vi "UHR-Fleezers Control (host) -TL FB Corrected Ronen semipassive - stepping.vi"(0 "Tab Control":T5(tab)=enum."Trap Control (RF)") -> ()   [LabVIEW 2013] (continued)
        n480 = xnode "Read/Write Control"("FPGA VI Reference In"=w830, "error in"=w829, "Phase count adjustment"=w826) -> ("FPGA VI Reference Out"=w825:T20, "error out"=w824:errorcluster)
        n481 = Or(x="- phase (AI1)", y="+ phase (AI1)") -> (x .or. y?=w821:bool)
        n482 = xnode "Read/Write Control"("FPGA VI Reference In"=w825, "error in"=w824, "+ phase"=w821) -> ("error out"=w820:errorcluster)  [unwired: 1 out]
      }
      event "Signals to Plot": Double Click {
        w833 = u32 9868950 ("Color Box")
        n483 = event-data() -> ("Row"=w835:i32)  [unwired: 9 out]
        n484 = property on="All Signals" class="WFChart (strict)"("Active Plot"=w835) -> (error out=w846:errorcluster)  [unwired: 2 in, 1 out]
        n485 = property on="All Signals" class="WFChart (strict)" props=["Plot", "Visible?", "Plot", "Plot Color"](error in=w846) -> (error out=w845:errorcluster, "Plot.Visible?"=w844:bool)  [unwired: 1 in, 2 out]
        n486 = Select(t=FALSE ("Plot.Visible"), s=w844, f=TRUE ("Plot.Visible")) -> (s? t:f=w839:bool)
        n487 = property on="All Signals" class="WFChart (strict)"(error in=w845, "Plot.Visible?"=w839) -> (error out=w841:errorcluster)  [unwired: 1 in, 1 out]
        n488 = property on="All Signals" class="WFChart (strict)"(error in=w841) -> (error out=w836:errorcluster, "Plot.Plot Color"=w840:u32)  [unwired: 1 in, 1 out]
        n489 = property on="Signals to Plot" class="LstBox (strict)"(error in=w836, "Active Row"=w835) -> (error out=w834:errorcluster)  [unwired: 1 in, 1 out]
        n490 = Select(t=w840, s=w839, f=u32 0) -> (s? t:f=w837:u32)
        n491 = property on="Signals to Plot" class="LstBox (strict)"(error in=w834, "CellFontColor"=w837, "SelColor"=w833, "CellBG"=w833, "CellFontSize"=u32 20 ("Active Row:Cell Font:Size"), "CellFontBold"=TRUE ("Active Row:Cell Font:Bold")) -> ()  [unwired: 1 in, 2 out]
      }
      event "Dynamic Force FB": Value Change {
        n492 = event-data() -> ()  [unwired: 7 out]
        n493 = xnode "Read/Write Control"("FPGA VI Reference In"=w848, "Dynamic Force FB (Ronen)"="Dynamic Force FB") -> ()  [unwired: 1 in, 2 out]
      }
      event "BD 1 Frequency 1 (MHz)", "BD 1 Frequency 2 (MHz)", "BD 1 Frequency 3 (MHz)", "BD 2 Frequency 1 (MHz)", "BD 2 Frequency 2 (MHz)", "BD 2 Frequency 3 (MHz)", "Trap Delta (MHz)": Value Change {
        # "anytime one of the frequencies is changed, write it to the RF board UNLESS Set 2 is being oscillated. The oscillation\nscript writes the frequencies to the RF board."
        n494 = event-data() -> ("CtlRef"=w851:refnum<vi>)  [unwired: 6 out]
        n495 = control-ref of="Trap Delta (MHz)"() -> (w850:refnum<vi>)
        n496 = Equal?(x=w850, y=w851) -> (x = y?=w849:bool)
        n497 = case shown="False" "Oscillate Set 2" {
          tunnel: w854 -> [w875 _]
          tunnel: [w874 w887] -> w853
          tunnel: w852 -> [w873 w887]
          tunnel: w849 -> [w860 _]
          frame False {
            n498 = case shown="False" "Symmetric manual \ntrap motion" {
              tunnel: [w880 w886] -> w861
              tunnel: "Trap Delta (MHz)" -> [w879 w885]
              tunnel: [w878 w882] -> w857
              frame False {
                w880 = 90.0
                n499 = Subtract(x=w880, y=w879) -> (x-y=w878:dbl)
              }
              frame True {
                w881 = 80
                n500 = Divide(x=w885, y=2) -> (x/y=w883:dbl)
                n501 = Subtract(x=w881, y=w883) -> (x-y=w882:dbl)
                n502 = Add(x=w881, y=w883) -> (x+y=w886:dbl)
              }
            }
            n503 = local read "BD 1 Frequency 2 (MHz)"() -> (w862:dbl)
            n504 = local write "BD 1 Frequency 1 (MHz)"(w857) -> ()
            n505 = Select(t=w861, s=w860, f=w862) -> (s? t:f=w859:dbl)
            n506 = local read "Y RF Frequency Limits (MHz)"() -> (w863:T17)
            n507 = local read "X RF Frequency Limits (MHz)"() -> (w864:T17)
            n508 = local read "BD 1 Frequency 3 (MHz)"() -> (w876:dbl)
            n509 = local write "BD 1 Frequency 2 (MHz)"(w859) -> ()
            n510 = local read "BD 2 Frequency 1 (MHz)"() -> (w867:dbl)
            n511 = local read "BD 2 Frequency 2 (MHz)"() -> (w866:dbl)
            n512 = local read "BD 2 Frequency 3 (MHz)"() -> (w877:dbl)
            n513 = call "set RF board frequency - interlace.vi"("Board 2 Frequency Limits"=w863, "Board 1 Frequency Limits"=w864, "error in"=w873, "FPGA VI Reference In"=w875, "Board 2 Frequency 3 (MHz)"=w877, "Board 1 Frequency 3 (MHz)"=w876, "Board 2 Frequency 2 (MHz)"=w866, "Board 2 Frequency 1 (MHz)"=w867, "Board 1 Frequency 2 (MHz)"=w859, "Board 1 Frequency 1  (MHz)"=w857) -> ("error out"=w874:errorcluster)  [unwired: 1 out]
            n514 = Subtract(x=w867, y=w866) -> (x-y=w871:dbl)
            n515 = Subtract(x=w859, y=w857) -> (x-y=w872:dbl)
            n516 = Square(x=w871) -> (x^2=w869:dbl)
            n517 = Square(x=w872) -> (x^2=w870:dbl)
            n518 = Add(x=w870, y=w869) -> (x+y=w868:dbl)
            n519 = Square Root(x=w868) -> (sqrt(x)=w865:dbl)
            n520 = local write "Trap Delta (MHz)"(w865) -> ()
            n521 = property on="Initial delta (MHz)" class="DigNum (strict)"("Val(Sgnl)"=w865) -> ()  [unwired: 2 in, 2 out]
          }
          frame True {
          }
        }
      }
      event "Round T1 X": Value Change {
        n522 = event-data() -> ()  [unwired: 7 out]
        n523 = local read "BD 1 Frequency 1 (MHz)"() -> (w890:dbl)
        n524 = Round To Nearest(number=w890) -> (nearest integer value=w889:dbl)
        n525 = property on="BD 1 Frequency 1 (MHz)" class="DigNum (strict)"("Val(Sgnl)"=w889) -> ()  [unwired: 2 in, 2 out]
      }
      event "Restart RF": Value Change {
        n526 = event-data() -> ()  [unwired: 7 out]
        n527 = xnode "Read/Write Control"("FPGA VI Reference In"=w928, "error in"=w923, "FPGA Controls  RF Box"=FALSE) -> ("FPGA VI Reference Out"=w927:T20, "error out"=w922:errorcluster)
        n528 = local read "Y RF Amplitude Limits (%)"() -> (w903:T17)
        n529 = local read "X RF Amplitude Limits (%)"() -> (w904:T17)
        n530 = local read "X RF Frequency Limits (MHz)"() -> (w906:T17)
        n531 = local read "Y RF Frequency Limits (MHz)"() -> (w905:T17)
        n532 = xnode "Read/Write Control"("FPGA VI Reference In"=w927, "error in"=w922, "Direct RF Box  Communication"=TRUE) -> ("FPGA VI Reference Out"=w926:T20, "error out"=w921:errorcluster)
        n533 = local read "BD 2 Frequency 3 (MHz)"() -> (w913:dbl)
        n534 = local read "BD 2 Frequency 2 (MHz)"() -> (w914:dbl)
        n535 = local read "BD 1 Frequency 3 (MHz)"() -> (w917:dbl)
        n536 = local read "BD 1 Frequency 1 (MHz)"() -> (w918:dbl)
        n537 = local read "BD 2 Frequency 1 (MHz)"() -> (w915:dbl)
        n538 = local read "BD 1 Frequency 2 (MHz)"() -> (w916:dbl)
        n539 = call "Initialize RF boards - interlace 3.vi"("error in"=w921, "FPGA VI Reference In"=w926) -> ("error out"=w920:errorcluster, "FPGA VI Reference Out"=w925:T20)
        n540 = local read "BD 2 Amplitude 2 (%)"() -> (w908:dbl)
        n541 = local read "BD 2 Amplitude 1 (%)"() -> (w909:dbl)
        n542 = local read "BD 2 Amplitude 3 (%)"() -> (w907:dbl)
        n543 = local read "BD 1 Amplitude 3 (%)"() -> (w912:dbl)
        n544 = local read "BD 1 Amplitude 1 (%)"() -> (w911:dbl)
        n545 = local read "BD 1 Amplitude 2 (%)"() -> (w910:dbl)
        n546 = call "set RF board frequency - interlace.vi"("Board 2 Frequency Limits"=w905, "Board 1 Frequency Limits"=w906, "error in"=w920, "FPGA VI Reference In"=w925, "Board 2 Frequency 3 (MHz)"=w913, "Board 1 Frequency 3 (MHz)"=w917, "Board 2 Frequency 2 (MHz)"=w914, "Board 2 Frequency 1 (MHz)"=w915, "Board 1 Frequency 2 (MHz)"=w916, "Board 1 Frequency 1  (MHz)"=w918) -> ("error out"=w919:errorcluster, "FPGA VI Reference Out"=w924:T20)
        n547 = call "set RF board amplitude - interlace.vi"("Board 2 Amplitude Limits"=w903, "Board 1 Amplitude Limits"=w904, "error in"=w919, "FPGA VI Reference In"=w924, "Board 2 Amplitude 3 (%)"=w907, "Board 1 Amplitude 3 (%)"=w912, "Board 2 Amplitude 2 (%)"=w908, "Board 2 Amplitude 1 (%)"=w909, "Board 1 Amplitude 2 (%)"=w910, "Board 1 Amplitude 1 (%)"=w911) -> ("error out"=w896:errorcluster, "FPGA VI Reference Out"=w900:T20)
        n548 = xnode "Read/Write Control"("FPGA VI Reference In"=w900, "error in"=w896, "Direct RF Box  Communication"=FALSE) -> ("FPGA VI Reference Out"=w899:T20, "error out"=w898:errorcluster)
        n549 = flat-sequence {
          tunnel: w898 -> [w929]
          tunnel: [w929] -> w897
          frame #0 {
            n550 = Wait (ms)(milliseconds to wait=u32 50) -> ()  [unwired: 1 out]
          }
        }
        n551 = xnode "Read/Write Control"("FPGA VI Reference In"=w899, "error in"=w897, "FPGA Controls  RF Box"=TRUE) -> ("error out"=w892:errorcluster)  [unwired: 1 out]
        n552 = property on="Restart RF" class="Bool (strict)"(error in=w892, "Value"=FALSE ("Restart RF")) -> (error out=w891:errorcluster)  [unwired: 1 in, 1 out]
      }
      event "Round T2 X": Value Change {
        n553 = event-data() -> ()  [unwired: 7 out]
        n554 = local read "BD 1 Frequency 2 (MHz)"() -> (w932:dbl)
        n555 = Round To Nearest(number=w932) -> (nearest integer value=w931:dbl)
        n556 = property on="BD 1 Frequency 2 (MHz)" class="DigNum (strict)"("Val(Sgnl)"=w931) -> ()  [unwired: 2 in, 2 out]
      }
      event "Stop All": Value Change {
        n557 = event-data() -> ()  [unwired: 7 out]
        n558 = call "hamilton_controller.vi"("action"=T21."DISCONNECT") -> ()  [unwired: 10 in, 1 out]
        n559 = local read "Stop All"() -> (w935:bool)
      }
      event "Delayed Interlace Start": Value Change {
        n560 = event-data() -> ()  [unwired: 7 out]
        n561 = flat-sequence {
          frame #0 {
            n562 = Multiply(x="Delay to Interlace (s)", y=1000.0) -> (x*y=w938:dbl)
            n563 = Wait (ms)(milliseconds to wait=w938) -> ()  [unwired: 1 out]
          }
          frame #1 {
            n564 = property on="Green laser mode" class="RadioBtnsControl (strict)"("Val(Sgnl)"=enum32{"Laser ON", "Laser OFF", "Interlace"}."Interlace" ("Value (Signaling)")) -> ()  [unwired: 2 in, 2 out]
          }
        }
      }
      event "BD 1 Amplitude 1 (%)", "BD 1 Amplitude 2 (%)", "BD 1 Amplitude 3 (%)", "BD 2 Amplitude 1 (%)", "BD 2 Amplitude 2 (%)", "BD 2 Amplitude 3 (%)", "Trap 1 ON", "Trap 2 ON", "Trap 3 ON", "Feedback On/Off", "All FB On/Off": Value Change {
        w962 = i16 1 ("f")
        n565 = event-data() -> ()  [unwired: 7 out]
        n566 = local write "Trap 1 (ON/OFF)"("Trap 1 ON") -> ()
        n567 = local write "Trap 2 (ON/OFF)"("Trap 2 ON") -> ()
        n568 = Boolean To (0,1)(Boolean="Trap 3 ON") -> (0, 1=w963:i16)
        n569 = Boolean To (0,1)(Boolean="Trap 1 ON") -> (0, 1=w964:i16)
        n570 = Boolean To (0,1)(Boolean="Trap 2 ON") -> (0, 1=w965:i16)
        n571 = Select(t=w965, s="Trap ON/OFF X or Y Amp?", f=w962) -> (s? t:f=w960:i16)
        n572 = Select(t=w964, s="Trap ON/OFF X or Y Amp?", f=w962) -> (s? t:f=w961:i16)
        n573 = Select(t=w963, s="Trap ON/OFF X or Y Amp?", f=w962) -> (s? t:f=w959:i16)
        n574 = Select(t=w962, s="Trap ON/OFF X or Y Amp?", f=w965) -> (s? t:f=w957:i16)
        n575 = Select(t=w962, s="Trap ON/OFF X or Y Amp?", f=w964) -> (s? t:f=w958:i16)
        n576 = Select(t=w962, s="Trap ON/OFF X or Y Amp?", f=w963) -> (s? t:f=w956:i16)
        n577 = And(x="All FB On/Off", y="Feedback On/Off") -> (x .and. y?=w954:cluster{"Set 1":bool, "Set 2":bool})
        n578 = local read "BD 1 Amplitude 1 (%)"() -> (w974:dbl)
        n579 = local read "BD 1 Amplitude 2 (%)"() -> (w973:dbl)
        n580 = local read "BD 1 Amplitude 3 (%)"() -> (w972:dbl)
        n581 = Unbundle By Name(w954) -> ("Set 1"=w949:bool, "Set 2"=w946:bool)
        n582 = local read "Y RF Amplitude Limits (%)"() -> (w942:T17)
        n583 = local read "X RF Amplitude Limits (%)"() -> (w943:T17)
        n584 = local read "BD 2 Amplitude 1 (%)"() -> (w975:dbl)
        n585 = local read "BD 2 Amplitude 2 (%)"() -> (w976:dbl)
        n586 = local read "BD 2 Amplitude 3 (%)"() -> (w977:dbl)
        n587 = And(x="Trap 2 ON", y=w946) -> (x .and. y?=w944:bool)
        n588 = And(x="Trap 1 ON", y=w949) -> (x .and. y?=w947:bool)
        n589 = Multiply(x=w961, y=w974) -> (x*y=w969:dbl)
        n590 = Multiply(x=w973, y=w960) -> (x*y=w967:dbl)
        n591 = Multiply(x=w972, y=w959) -> (x*y=w968:dbl)
        n592 = Multiply(x=w975, y=w958) -> (x*y=w978:dbl)
        n593 = Multiply(x=w976, y=w957) -> (x*y=w979:dbl)
        n594 = Multiply(x=w977, y=w956) -> (x*y=w980:dbl)
        n595 = call "set RF board amplitude - interlace.vi"("Board 2 Amplitude Limits"=w942, "Board 1 Amplitude Limits"=w943, "error in"=w970, "FPGA VI Reference In"=w971, "Board 2 Amplitude 3 (%)"=w980, "Board 1 Amplitude 3 (%)"=w968, "Board 2 Amplitude 2 (%)"=w979, "Board 2 Amplitude 1 (%)"=w978, "Board 1 Amplitude 2 (%)"=w967, "Board 1 Amplitude 1 (%)"=w969) -> ("error out"=w951:errorcluster, "FPGA VI Reference Out"=w952:T20)
        n596 = xnode "Read/Write Control"("FPGA VI Reference In"=w952, "error in"=w951, "FB On/Off Set 1"=w947, "FB On/Off Set 2"=w944) -> ("error out"=w950:errorcluster)  [unwired: 1 out]
      }
      event "Load parameters": Value Change {
        n597 = event-data() -> ()  [unwired: 7 out]
        n598 = property on="Saved AOD Raster Scan Parameter Sets" class="Arr (strict)"() -> ("Index Values"=w991:u32[])  [unwired: 2 in, 2 out]
        n599 = Index Array(array=w991, index=0) -> (element=w988:u32)
        n600 = local write "Load parameters"(FALSE ("Load parameters")) -> ()
        n601 = Index Array(array="Saved AOD Raster Scan Parameter Sets", index=w988) -> (element=w987:T31)
        n602 = Unbundle By Name(w987) -> ("Scan Range AOD (nm) 2"=w986:dbl, "Step Size AOD (nm) 2"=w985:dbl, "Scan Speed AOD (nm/s) 2"=w984:dbl, "Number of scans (AOD) 2"=w983:u16)
        n603 = flat-sequence {
          tunnel: w986 -> [w994]
          tunnel: w985 -> [w993]
          tunnel: w984 -> [w992]
          tunnel: w983 -> [w995]
          frame #0 {
            n604 = local write "Scan Speed (nm/s)"(w992) -> ()
            n605 = local write "Scan Range (nm)"(w994) -> ()
            n606 = local write "Step Size (nm)"(w993) -> ()
          }
          frame #1 {
            n607 = property on="Number of F/B Scans (AOD)" class="DigNum (strict)"("Val(Sgnl)"=w995) -> ()  [unwired: 2 in, 2 out]
          }
        }
      }
      event "Trap 1 (ON/OFF)", "Trap 2 (ON/OFF)": Value Change {
        n608 = event-data() -> ()  [unwired: 7 out]
        n609 = property on="Trap 2 ON" class="Bool (strict)"("Val(Sgnl)"="Trap 2 (ON/OFF)") -> ()  [unwired: 2 in, 2 out]
        n610 = property on="Trap 1 ON" class="Bool (strict)"("Val(Sgnl)"="Trap 1 (ON/OFF)") -> ()  [unwired: 2 in, 2 out]
      }
      event "DIO count 1 (ticks)", "DIO count 2 (ticks)", "DIO count 3 (ticks)", "Interlace", "Number Interlace Sets", "Not-Interlacing Set": Value Change {
        n611 = event-data() -> ()  [unwired: 7 out]
        n612 = local read "DIO count 3 (ticks)"() -> (w1008:u32)
        n613 = local read "DIO count 1 (ticks)"() -> (w1010:u32)
        n614 = local read "DIO count 2 (ticks)"() -> (w1009:u32)
        n615 = To Unsigned Byte Integer(number="Not-Interlacing Set") -> (unsigned 8bit integer=w999:u8)
        n616 = Add(x=w999, y=u8 1) -> (x+y=w1003:u8)
        n617 = xnode "Read/Write Control"("FPGA VI Reference In"=w1014, "error in"=w1012, "DIO count 1 (ticks)"=w1010, "DIO count 2 (ticks)"=w1009, "DIO count 3 (ticks)"=w1008, "Interlace ON/OFF"="Interlace", "Number Interlace Cycles"="Number Interlace Sets", "Interlace Off Parameters"=w1003) -> ("error out"=w1013:errorcluster)  [unwired: 1 out]
        n618 = Build Array(w1010, w1009, w1008) -> (w1001:u32[])
        n619 = Split 1D Array(array=w1001, index="Number Interlace Sets") -> (first subarray=w1011:u32[])  [unwired: 1 out]
        n620 = Index Array(array=w1001, index=w999) -> (element=w1000:u32)
        n621 = Add Array Elements(numeric array=w1011) -> (sum=w1005:u32)
        n622 = Select(t=w1005, s="Interlace", f=w1000) -> (s? t:f=→"Total Counts (ticks)":u32)
      }
      event "Reset Feedback": Value Change {
        n623 = event-data() -> ()  [unwired: 7 out]
        n624 = Unbundle By Name("Reset Feedback") -> ("Set 1"=w1018:bool, "Set 2"=w1017:bool)
        n625 = xnode "Read/Write Control"("FPGA VI Reference In"=w1020, "error in"=w1015, "FB Reset Set 1"=w1018, "FB Reset Set 2"=w1017) -> ("error out"=w1016:errorcluster)  [unwired: 1 out]
      }
      event "PID Gains": Value Change {
        n626 = event-data() -> ()  [unwired: 7 out]
        n627 = Unbundle By Name("PID Gains") -> ("Set 1"=w1024:T15, "Set 2"=w1023:T15)
        n628 = xnode "Read/Write Control"("FPGA VI Reference In"=w1025, "error in"=w1021, "FB Gains Set 1"=w1024, "FB Gains Set 2"=w1023) -> ("error out"=w1022:errorcluster)  [unwired: 1 out]
      }
      event "AI2 to Setpoint", "Trap Intensity\nSetpoints (V)": Value Change {
        n629 = event-data() -> ()  [unwired: 7 out]
        n630 = xnode "Read/Write Control"("FPGA VI Reference In"=w1031, "error in"=w1027) -> ("FPGA VI Reference Out"=w1030:T20, "error out"=w1029:errorcluster, "AI4 Y Sum Set 1"=w1038, "AI4 Y Sum Set 2"=w1037)
        n631 = Cluster To Array(cluster="AI2 to Setpoint") -> (array=w1041:bool[])
        n632 = local read "AI2 (V)"() -> (w1039:cluster{"Set 1":dbl, "Set 2":dbl})
        n633 = Or Array Elements(Boolean array=w1041) -> (logical OR=w1042:bool)
        n634 = Bundle By Name(cluster=w1039, "Set 1"=w1038, "Set 2"=w1037) -> (w1036:cluster{"Set 1":dbl, "Set 2":dbl})
        n635 = Divide(x=w1036, y=3276.7) -> (x/y=w1035:cluster{"Set 1":dbl, "Set 2":dbl})
        "AI2 (V)" <- w1035
        n636 = case shown="True" w1042 {
          tunnel: [w1045 w1062] -> w1034
          tunnel: "AI2 to Setpoint" -> [_ w1058]
          tunnel: "Trap Intensity\nSetpoints (V)" -> [w1046 w1061]
          tunnel: w1035 -> [_ w1055]
          frame False {
            n637 = Multiply(x=3276.7, y=w1046) -> (x*y=w1047:cluster{"Set 1":dbl, "Set 2":dbl})
            n638 = To Word Integer(number=w1047) -> (16bit integer=w1045:cluster{"Set 1":i16, "Set 2":i16})
          }
          frame True {
            n639 = Unbundle By Name(w1055) -> ("Set 1"=w1054:dbl, "Set 2"=w1053:dbl)
            n640 = Unbundle By Name(w1061) -> ("Set 1"=w1060:dbl, "Set 2"=w1059:dbl)
            n641 = Unbundle By Name(w1058) -> ("Set 1"=w1057:bool, "Set 2"=w1056:bool)
            n642 = Select(t=w1054, s=w1057, f=w1060) -> (s? t:f=w1052:dbl)
            n643 = Select(t=w1053, s=w1056, f=w1059) -> (s? t:f=w1051:dbl)
            n644 = Bundle By Name(cluster=w1061, "Set 1"=w1052, "Set 2"=w1051) -> (w1049:cluster{"Set 1":dbl, "Set 2":dbl})
            n645 = local write "Trap Intensity\nSetpoints (V)"(w1049) -> ()
            n646 = Multiply(x=3276.7, y=w1049) -> (x*y=w1050:cluster{"Set 1":dbl, "Set 2":dbl})
            n647 = To Word Integer(number=w1050) -> (16bit integer=w1062:cluster{"Set 1":i16, "Set 2":i16})
          }
        }
        n648 = Unbundle By Name(w1034) -> ("Set 1"=w1033:i16, "Set 2"=w1032:i16)
        n649 = xnode "Read/Write Control"("FPGA VI Reference In"=w1030, "error in"=w1029, "FB Setpoint Set 1"=w1033, "FB Setpoint Set 2"=w1032) -> ("error out"=w1028:errorcluster)  [unwired: 1 out]
      }
      event "Invert GI": Value Change {
        n650 = event-data() -> ()  [unwired: 7 out]
        n651 = xnode "Read/Write Control"("FPGA VI Reference In"=w1067, "error in"=w1065, "Invert GI"="Invert GI", "Invert GI 2"="Invert GI") -> ("error out"=w1066:errorcluster)  [unwired: 1 out]
      }
      event "Green FB Setpoint (mV)", "Green FB Gains", "Green FB On/Off", "Current When FB OFF (%)", "Green int current ON count adj": Value Change {
        n652 = event-data() -> ()  [unwired: 7 out]
        n653 = local read "Green FB Setpoint (mV)"() -> (w1074:dbl)
        n654 = local read "Current When FB OFF (%)"() -> (w1077:dbl)
        n655 = Multiply(x=w1074, y=3.2767) -> (x*y=w1073:dbl)
        n656 = Multiply(x=w1077, y=655.35) -> (x*y=w1078:dbl)
        n657 = To Unsigned Word Integer(number=w1078) -> (unsigned 16bit integer=w1076:u16)
        n658 = local read "Green int current ON count adj"() -> (w1081:u32)
        n659 = local read "Green FB Gains"() -> (w1080:T15)
        n660 = local read "Green Laser ON/Interlacing"() -> (w1071:bool)
        n661 = local read "Green laser mode"() -> (w1070:enum32{"Laser ON", "Laser OFF", "Interlace"})
        n662 = local read "Green FB On/Off"() -> (w1082:bool)
        n663 = Equal?(x=w1070, y=enum32{"Laser ON", "Laser OFF", "Interlace"}."Interlace") -> (x = y?=w1068:bool)
        n664 = Compound Arithmetic op=AND(w1068, w1082, w1071) -> (w1072:bool)
        n665 = xnode "Read/Write Control"("FPGA VI Reference In"=w1085, "error in"=w1084, "Green FB Setpoint"=w1073, "Green FB On/Off"=w1072, "Current Out"=w1076, "Green int current ON count adj"=w1081, "Green FB Gains"=w1080) -> ("error out"=w1083:errorcluster)  [unwired: 1 out]
      }
      event "Green laser mode", "Green Laser ON/Interlacing": Value Change {
        n666 = event-data() -> ()  [unwired: 7 out]
        n667 = case shown="True" "Green Laser ON/Interlacing" {
          tunnel: "Green laser mode" -> [_ w1099]
          tunnel: [enum32{"Laser ON", "Laser OFF", "Interlace"}."Laser OFF" ("Green laser mode") w1099] -> w1087
          tunnel: [FALSE w1095] -> w1086
          frame False {
          }
          frame True {
            n668 = local read "Green FB On/Off"() -> (w1096:bool)
            n669 = Equal?(x=w1099, y=enum32{"Laser ON", "Laser OFF", "Interlace"}."Interlace") -> (x = y?=w1097:bool)
            n670 = And(x=w1097, y=w1096) -> (x .and. y?=w1095:bool)
          }
        }
        n671 = xnode "Read/Write Control"("FPGA VI Reference In"=w1092, "error in"=w1090, "Operating Mode"=w1087, "Operating Mode 2"=w1087, "Green FB On/Off"=w1086) -> ("error out"=w1091:errorcluster)  [unwired: 1 out]
      }
      event "- phase (APD 1 Gate)", "+ phase (APD 1 Gate)": Value Change {
        n672 = event-data() -> ()  [unwired: 7 out]
        n673 = local read "Phase Adj. (APD 1 Gate)"() -> (w1100:i16)
        n674 = Negate(x=w1100) -> (-x=w1108:i16)
        n675 = Select(t=w1108, s="- phase (APD 1 Gate)", f=w1100) -> (s? t:f=w1107:i16)
        n676 = Or(x="- phase (APD 1 Gate)", y="+ phase (APD 1 Gate)") -> (x .or. y?=w1103:bool)
        n677 = xnode "Read/Write Control"("FPGA VI Reference In"=w1110, "error in"=w1109, "Phase count adjustment (APD 1 Gate)"=w1107) -> ("FPGA VI Reference Out"=w1105:T20, "error out"=w1106:errorcluster)
        n678 = xnode "Read/Write Control"("FPGA VI Reference In"=w1105, "error in"=w1106, "+ phase (APD 1 Gate)"=w1103) -> ("error out"=w1104:errorcluster)  [unwired: 1 out]
      }
      event "+ phase (APD 2 Gate)", "- phase (APD 2 Gate)": Value Change {
        n679 = event-data() -> ()  [unwired: 7 out]
        n680 = local read "Phase Adj. (APD 2 Gate)"() -> (w1111:i16)
        n681 = Negate(x=w1111) -> (-x=w1119:i16)
        n682 = Select(t=w1119, s="- phase (APD 2 Gate)", f=w1111) -> (s? t:f=w1118:i16)
        n683 = Or(x="- phase (APD 2 Gate)", y="+ phase (APD 2 Gate)") -> (x .or. y?=w1114:bool)
        n684 = xnode "Read/Write Control"("FPGA VI Reference In"=w1121, "error in"=w1120, "Phase count adjustment (APD 2 Gate)"=w1118) -> ("FPGA VI Reference Out"=w1116:T20, "error out"=w1117:errorcluster)
        n685 = xnode "Read/Write Control"("FPGA VI Reference In"=w1116, "error in"=w1117, "+ phase (APD 2 Gate)"=w1114) -> ("error out"=w1115:errorcluster)  [unwired: 1 out]
      }
      event "Phase Adj. (APD Acq)", "+ phase (APD Acq)", "- phase (APD Acq)": Value Change {
        n686 = event-data() -> ()  [unwired: 7 out]
        n687 = local read "Phase Adj. (APD Acq)"() -> (w1124:i16)
        n688 = Negate(x=w1124) -> (-x=w1130:i16)
        n689 = Select(t=w1130, s="+ phase (APD Acq)", f=w1124) -> (s? t:f=w1129:i16)
        n690 = Or(x="+ phase (APD Acq)", y="- phase (APD Acq)") -> (x .or. y?=w1125:bool)
        n691 = xnode "Read/Write Control"("FPGA VI Reference In"=w1132, "error in"=w1131, "Phase Count Adjustment (APD Acq)"=w1129) -> ("FPGA VI Reference Out"=w1127:T20, "error out"=w1128:errorcluster)
        n692 = xnode "Read/Write Control"("FPGA VI Reference In"=w1127, "error in"=w1128, "+ phase (APD Acq)"=w1125) -> ("error out"=w1126:errorcluster)  [unwired: 1 out]
      }
      event "Phase adj. (GI)", "+ phase (GI)", "- phase (GI)": Value Change {
        n693 = event-data() -> ()  [unwired: 7 out]
        n694 = Negate(x="Phase adj. (GI)") -> (-x=w1141:i16)
        n695 = Select(t=w1141, s="+ phase (GI)", f="Phase adj. (GI)") -> (s? t:f=w1140:i16)
        n696 = Or(x="+ phase (GI)", y="- phase (GI)") -> (x .or. y?=w1136:bool)
        n697 = xnode "Read/Write Control"("FPGA VI Reference In"=w1143, "error in"=w1142, "Phase count adjustment (GI)"=w1140) -> ("FPGA VI Reference Out"=w1138:T20, "error out"=w1139:errorcluster)
        n698 = xnode "Read/Write Control"("FPGA VI Reference In"=w1138, "error in"=w1139, "+ phase (GI)"=w1136) -> ("error out"=w1137:errorcluster)  [unwired: 1 out]
      }
      event "Phase adj. (GI) 2", "+ phase (GI) 2", "- phase (GI) 2": Value Change {
        n699 = event-data() -> ()  [unwired: 7 out]
        n700 = Negate(x="Phase adj. (GI) 2") -> (-x=w1152:i16)
        n701 = Select(t=w1152, s="+ phase (GI) 2", f="Phase adj. (GI) 2") -> (s? t:f=w1151:i16)
        n702 = Or(x="+ phase (GI) 2", y="- phase (GI) 2") -> (x .or. y?=w1147:bool)
        n703 = xnode "Read/Write Control"("FPGA VI Reference In"=w1154, "error in"=w1153, "Phase count adjustment (GI) 2"=w1151) -> ("FPGA VI Reference Out"=w1149:T20, "error out"=w1150:errorcluster)
        n704 = xnode "Read/Write Control"("FPGA VI Reference In"=w1149, "error in"=w1150, "+ phase (GI) 2"=w1147) -> ("error out"=w1148:errorcluster)  [unwired: 1 out]
      }
      event "Phase adj. (Green FB)", "- phase (Green FB)", "+ phase (Green FB)": Value Change {
        n705 = event-data() -> ()  [unwired: 7 out]
        n706 = Negate(x="Phase adj. (Green FB)") -> (-x=w1163:i16)
        n707 = Select(t=w1163, s="+ phase (Green FB)", f="Phase adj. (Green FB)") -> (s? t:f=w1162:i16)
        n708 = Or(x="+ phase (Green FB)", y="- phase (Green FB)") -> (x .or. y?=w1158:bool)
        n709 = xnode "Read/Write Control"("FPGA VI Reference In"=w1165, "error in"=w1164, "Phase count adjustment (Green FB)"=w1162) -> ("FPGA VI Reference Out"=w1160:T20, "error out"=w1161:errorcluster)
        n710 = xnode "Read/Write Control"("FPGA VI Reference In"=w1160, "error in"=w1161, "+ phase (Green FB)"=w1158) -> ("error out"=w1159:errorcluster)  [unwired: 1 out]
      }
      event "Invert APD Gate", "APD Gate ON Count", "APD Gate OFF Count", "APD Gate", "APD Integration Time (s)", "APD 1 AO Mult.", "APD 2 AO Mult.": Value Change {
        n711 = event-data() -> ()  [unwired: 7 out]
        n712 = local read "APD Integration Time (s)"() -> (w1166:dbl)
        n713 = local read "APD Gate ON Count"() -> (w1179:u32)
        n714 = local read "APD Gate OFF Count"() -> (w1178:u32)
        n715 = local read "Invert APD Gate"() -> (w1180:bool)
        n716 = local read "APD Gate"() -> (w1177:enum32{"ON", "OFF", "Interlace"})
        n717 = Multiply(x=w1166, y=40000000.0) -> (x*y=w1175:dbl)
        n718 = Reciprocal(x=w1166) -> (1/x=→"APD Acq Rate (Hz)":dbl)
        n719 = To Unsigned Long Integer(number=w1175) -> (unsigned 32bit integer=w1174:u32)
        n720 = local read "DMA Update Period (s)"() -> (w1167:dbl)
        n721 = Divide(x=w1167, y=w1166) -> (x/y=w1170:dbl)
        n722 = local read "APD 1 AO Mult."() -> (w1172:i16)
        n723 = local read "APD 2 AO Mult."() -> (w1171:i16)
        n724 = Multiply(x=2.0, y=w1170) -> (x*y=w1169:dbl)
        n725 = local write "APD Samples/FIFO Acq."(w1170) -> ()
        n726 = local write "APD Elements/DMA read"(w1169) -> ()
        n727 = xnode "Read/Write Control"("FPGA VI Reference In"=w1183, "error in"=w1182, "Invert APD Gate"=w1180, "APD Gate ON Count"=w1179, "APD Gate OFF Count"=w1178, "APD Acq Rate Count"=w1174, "APD Gate Operating Mode"=w1177, "APD 1 AO scale factor"=w1172, "APD 2 AO scale factor"=w1171) -> ("error out"=w1181:errorcluster)  [unwired: 1 out]
      }
      event "GI Frequency, ON count", "Green FB Count", "GI Frequency, OFF count": Value Change {
        n728 = event-data() -> ()  [unwired: 7 out]
        n729 = xnode "Read/Write Control"("FPGA VI Reference In"=w1189, "error in"=w1187, "Green interlace ON count"="GI Frequency, ON count", "Green interlace OFF count"="GI Frequency, OFF count", "Green interlace ON count 2"="GI Frequency, ON count", "Green interlace OFF count 2"="GI Frequency, OFF count", "Green FB Count"="Green FB Count") -> ("error out"=w1188:errorcluster)  [unwired: 1 out]
      }
      event "Number of F/B Scans (AOD)", "Scan Speed (nm/s)", "Scan BD", "Initial delta (MHz)", "Step Size (nm)", "Scan Range (nm)": Value Change {
        w1251 = 123.0  # AOM cal (nm/MHz)
        n730 = event-data() -> ()  [unwired: 7 out]
        n731 = local read "BD 1 Frequency 1 (MHz)"() -> (w1234:dbl)
        n732 = local read "AOM X Cal (nm/MHz)"() -> (w1226:dbl)
        n733 = local read "X RF Frequency Limits (MHz)"() -> (w1238:T17)
        n734 = local read "Y RF Frequency Limits (MHz)"() -> (w1235:T17)
        n735 = local read "BD 2 Frequency 1 (MHz)"() -> (w1240:dbl)
        n736 = Negate(x="Scan Range (nm)") -> (-x=w1204:dbl)
        n737 = Divide(x=w1204, y=w1226) -> (x/y=w1208:dbl)
        n738 = Select(t=w1238, s="Scan BD", f=w1235) -> (s? t:f=w1237:T17)
        n739 = Select(t=w1234, s="Scan BD", f=w1240) -> (s? t:f=w1239:dbl)
        n740 = Unbundle By Name(w1237) -> ("Maximum"=w1246:dbl, "Minimum"=w1245:dbl)
        n741 = Add(x=w1208, y=w1239) -> (x+y=w1243:dbl)
        n742 = Divide(x=w1204, y="Step Size (nm)") -> (x/y=w1223:dbl)
        n743 = Divide(x="Step Size (nm)", y=w1226) -> (x/y=w1232:dbl)
        n744 = Absolute Value(x=w1223) -> (abs(x)=w1207:dbl)
        n745 = Sign(1:w1204) -> (0:w1205:dbl)
        n746 = In Range and Coerce(upper limit=w1246, x=w1243, lower limit=w1245) -> (coerced(x)=w1242:dbl, In Range?=w1244:bool)
        n747 = To Unsigned Quad Integer(1:w1207) -> (0:w1222:u64)
        "Scan steps (AOD)" <- w1222
        n748 = call "IR AOM freq to word.vi"("Frequency In (MHz)"=w1232) -> ("Frequency Word Out (double)"=w1229:dbl)
        n749 = Multiply(x=w1205, y=w1229) -> (x*y=w1206:dbl)
        n750 = Subtract(x=w1243, y=w1242) -> (x-y=w1241:dbl)
        n751 = To Quad Integer(1:w1206) -> (0:w1228:i64)
        "Incr. int (AOD)" <- w1228
        n752 = Subtract(x=w1208, y=w1241) -> (x-y=w1227:dbl)
        "Scan Range (MHz)" <- w1227
        n753 = Select(t=w1208, s=w1244, f=w1227) -> (s? t:f=w1247:dbl)
        n754 = Multiply(x=w1227, y=w1226) -> (x*y=w1225:dbl)
        n755 = Decrement(x=w1222) -> (x-1=w1275:u64)
        n756 = Negate(x=w1225) -> (-x=w1221:dbl)
        n757 = local write "Scan Range (nm)"(w1221) -> ()
        n758 = Divide(x=w1247, y=w1275) -> (x/y=w1231:dbl)
        "Scan Increment (MHz)" <- w1231
        n759 = call "IR AOM freq to word.vi"("Frequency In (MHz)"=w1231) -> ("Frequency Word Out (double)"=w1230:dbl)
        n760 = Divide(x="Step Size (nm)", y="Scan Speed (nm/s)") -> (x/y=w1218:dbl)
        n761 = To Quad Integer(1:w1230) -> ()  [unwired: 1 out]
        n762 = local read "Number Interlace Sets"() -> (w1202:u8)
        n763 = local read "AI Count (ticks)"() -> (w1203:u32)
        n764 = local read "Total Counts (ticks)"() -> (w1201:u32)
        n765 = local read "# Samples/trap"() -> (w1233:u32)
        n766 = Multiply(x=w1203, y=w1202) -> (x*y=w1200:u32)
        n767 = Divide(x=w1201, y=w1200) -> (x/y=w1199:dbl)
        n768 = Select(t=w1234, s="Scan BD", f=w1240) -> (s? t:f=w1272:dbl)
        "Initial freq. (MHz)" <- w1272
        n769 = Add(x=w1247, y=w1272) -> (x+y=→"Final freq. (MHz)":dbl)
        n770 = Divide(x=w1201, y=40000000.0) -> (x/y=w1217:dbl)
        n771 = Divide(x=w1218, y=w1217) -> (x/y=w1216:dbl)
        n772 = To Unsigned Quad Integer(1:w1216) -> (0:w1191:u64)
        n773 = Quotient & Remainder(x=w1191, y=u64 2) -> (x-y*floor(x/y)=w1195:u64)  [unwired: 1 out]
        n774 = Equal?(x=w1195, y=u64 0) -> (x = y?=w1193:bool)
        n775 = Decrement(x=w1191) -> (x-1=w1192:u64)
        n776 = Select(t=w1191, s=w1193, f=w1192) -> (s? t:f=w1190:u64)
        "Cycles/step (AOD)" <- w1190
        n777 = xnode "Read/Write Control"("FPGA VI Reference In"=w1283, "error in"=w1282, "Scan steps"=w1222, "Number of scans"="Number of F/B Scans (AOD)", "Cycles per step"=w1190, "Scan freq.  increment"=w1228, "Scan BD"="Scan BD") -> ("error out"=w1281:errorcluster)  [unwired: 1 out]
        n778 = Multiply(x=w1222, y=w1190) -> (x*y=w1276:u64)
        n779 = Multiply(x=w1276, y=u64 2) -> (x*y=w1198:u64)
        n780 = Multiply(x=w1199, y=w1198) -> (x*y=w1197:dbl)
        "Data points/scan (f/b)" <- w1197
        n781 = Multiply(x=w1197, y="Number of F/B Scans (AOD)") -> (x*y=w1279:dbl)
        "Data points/scans" <- w1279
        n782 = Divide(x=w1279, y=w1233) -> (x/y=→"N sets should be saved":dbl)
        n783 = Multiply(x=w1276, y=w1217) -> (x*y=w1215:dbl)
        "Time/Scan (s) (AOD)" <- w1215
        n784 = Select(t=w1247, s="Scan BD", f=0.0) -> (s? t:f=w1273:dbl)
        n785 = Select(t=0.0, s="Scan BD", f=w1247) -> (s? t:f=w1269:dbl)
        n786 = local read "BD 2 Frequency 2 (MHz)"() -> (w1265:dbl)
        n787 = local read "BD 1 Frequency 2 (MHz)"() -> (w1268:dbl)
        n788 = Add(x=w1269, y=w1240) -> (x+y=w1266:dbl)
        n789 = Add(x=w1234, y=w1273) -> (x+y=w1267:dbl)
        n790 = Multiply(x=w1215, y=2.0) -> (x*y=w1214:dbl)
        n791 = Multiply(x=w1214, y="Number of F/B Scans (AOD)") -> (x*y=w1211:dbl)
        n792 = Divide(x=w1211, y=60.0) -> (x/y=→"Time to Finish All (min)":dbl)
        n793 = Add(x="Trap 2 Bead Size (nm)", y="Trap 1 Bead Size (nm)") -> (x+y=w1255:dbl)
        n794 = local read "Initial delta (MHz)"() -> (w1252:dbl)
        n795 = Divide(x=w1255, y=2.0) -> (x/y=w1249:dbl)
        n796 = Subtract(x=w1266, y=w1265) -> (x-y=w1263:dbl)
        n797 = Subtract(x=w1267, y=w1268) -> (x-y=w1264:dbl)
        n798 = Square(x=w1263) -> (x^2=w1262:dbl)
        n799 = Square(x=w1264) -> (x^2=w1261:dbl)
        n800 = Add(x=w1261, y=w1262) -> (x+y=w1260:dbl)
        n801 = Square Root(x=w1260) -> (sqrt(x)=w1259:dbl)
        "Final delta (MHz)" <- w1259
        n802 = Multiply(x=w1251, y=w1259) -> (x*y=w1258:dbl)
        n803 = Multiply(x=w1252, y=w1251) -> (x*y=w1250:dbl)
        n804 = Subtract(x=w1250, y=w1249) -> (x-y=→"Initial sep (nm)":dbl)
        n805 = Subtract(x=w1258, y=w1249) -> (x-y=→"Final sep (nm)":dbl)
      }
      event "Raster Scanning...": Value Change {
        n806 = event-data() -> ("NewVal"=w1284:bool)  [unwired: 6 out]
        n807 = case shown="True" w1284 {
          frame False {
          }
          frame True {
            n808 = property on="BD 1 Frequency 1 (MHz)" class="DigNum (strict)"("Val(Sgnl)"=65.0 ("Value (Signaling)")) -> ()  [unwired: 2 in, 2 out]
          }
        }
      }
      event "Freq or Amp switch first", "Swap F1 and F2", "Freq switch delay", "Amp switch delay": Value Change {
        n809 = event-data() -> ()  [unwired: 7 out]
        n810 = local read "Freq or Amp switch first"() -> (w1286:bool)
        n811 = local read "Amp switch delay"() -> (w1287:u16)
        n812 = local read "Freq switch delay"() -> (w1289:u16)
        n813 = local read "Swap F1 and F2"() -> (w1288:bool)
        n814 = xnode "Read/Write Control"("FPGA VI Reference In"=w1292, "error in"=w1291, "Freq switch delay"=w1289, "Swap F1 and F2"=w1288, "Amp switch delay"=w1287, "Freq or Amp switch first"=w1286) -> ("error out"=w1290:errorcluster)  [unwired: 1 out]
      }
      event "Scan steps (MCL)", "Number of scans (MCL)", "Scan Range (V)\n(of steps)", "2D or 1D Scan", "N APD Samp/step", "Fast Scan Dir", "Continuous MCL Scanning", "Scan lines (y)": Value Change {
        w1294 = 32767.0 ("y")
        n815 = event-data() -> ()  [unwired: 7 out]
        n816 = Select(t="Scan lines (y)", s="2D or 1D Scan", f="Number of scans (MCL)") -> (s? t:f=w1299:u64)
        n817 = Decrement(x="Scan steps (MCL)") -> (x-1=w1315:u64)
        n818 = Divide(x="Scan Range (V)\n(of steps)", y=w1315) -> (x/y=w1314:dbl)
        "Desired Scan Incr (V)" <- w1314
        n819 = local read "APD Integration Time (s)"() -> (w1307:dbl)
        n820 = Multiply(x=w1314, y=w1294) -> (x*y=w1323:dbl)
        n821 = Divide(x=w1323, y=10.0) -> (x/y=w1313:dbl)
        "Desired incr (int)" <- w1313
        n822 = local read "Update Count (MCL)"() -> (w1319:u32)
        n823 = Round Toward -Infinity(1:w1313) -> (0:w1322:dbl)
        n824 = To Word Integer(number=w1322) -> (16bit integer=w1297:i16)
        "Actual Incr. int (MCL)" <- w1297
        n825 = Multiply(x=w1307, y=40000000.0) -> (x*y=w1320:dbl)
        n826 = Divide(x=w1320, y=w1319) -> (x/y=w1318:dbl)
        n827 = Multiply(x=i16 10, y=w1297) -> (x*y=w1295:i16)
        n828 = Multiply(x="N APD Samp/step", y=w1318) -> (x*y=w1317:dbl)
        "Cycles/step (MCL)" <- w1317
        n829 = Divide(x=w1295, y=w1294) -> (x/y=→"Actual MCL Inc (V)":dbl)
        n830 = Multiply(x="N APD Samp/step", y="Scan steps (MCL)") -> (x*y=w1309:dbl)
        n831 = local read "APD Samples/FIFO Acq."() -> (w1306:dbl)
        n832 = Multiply(x=w1309, y=u64 2) -> (x*y=w1308:dbl)
        "Data points/scan (f+b)" <- w1308
        n833 = Multiply(x=w1308, y=w1299) -> (x*y=w1326:dbl)
        "Data points/scans (MCL)" <- w1326
        n834 = Multiply(x=w1307, y=w1308) -> (x*y=w1300:dbl)
        "Time/f+b scan (s) (MCL)" <- w1300
        n835 = Divide(x=w1326, y=w1306) -> (x/y=→"N sets should be saved (MCL)":dbl)
        n836 = Multiply(x=w1300, y=w1299) -> (x*y=→"Total Time (s)":dbl)
        n837 = Not(x="Fast Scan Dir") -> (.not. x?=w1304:bool)
        n838 = xnode "Read/Write Control"("FPGA VI Reference In"=w1330, "error in"=w1329, "Scan steps (MCL)"="Scan steps (MCL)", "Number of scans (MCL)"=w1299, "Cycles per step (MCL)"=w1317, "Scan freq.  increment (MCL)"=w1297, "1D or 2D Scan?"="2D or 1D Scan", "MCL Scan Axis"=w1304, "Cont. Scan (MCL)"="Continuous MCL Scanning") -> ("error out"=w1328:errorcluster)  [unwired: 1 out]
      }
      event "Read Cal": Value Change {
        w1363 = 1000.0 ("y")
        w1351 = T30."big-endian, network order" ("byte order (0:big-endian, network order)")
        w1352 = -1 ("count (1)")
        n839 = event-data() -> ()  [unwired: 7 out]
        n840 = local read "Save file name"() -> (w1381:path)
        n841 = local write "Read Cal"(FALSE ("Read Cal")) -> ()
        n842 = Strip Path(path=w1381) -> (stripped path=w1380:path)  [unwired: 1 out]
        n843 = Path To String(path=w1380) -> (string=w1361:string)
        n844 = Concatenate Strings(w1361, "\\current.off" ("string")) -> (w1359:string)
        n845 = Concatenate Strings(w1361, "\\current.cal" ("string")) -> (w1378:string)
        n846 = String To Path(string=w1378) -> (path=w1377:path)
        n847 = String To Path(string=w1359) -> (path=w1358:path)
        n848 = Open/Create/Replace File(file path (use dialog)=w1377, operation (0:open)=T24."open", access (0:read/write)=enum16{"read/write", "read-only", "write-only"}."read-only") -> (refnum out=w1384:refnum<file>, error out=w1373:errorcluster)  [unwired: 1 in, 3 out]
        n849 = Deny Access(4:w1373, 7:w1384) -> (0:w1372:errorcluster, 3:w1376:refnum<file>)  [unwired: 1 out]
        n850 = Open/Create/Replace File(file path (use dialog)=w1358, operation (0:open)=T24."open", access (0:read/write)=enum16{"read/write", "read-only", "write-only"}."read-only") -> (refnum out=w1355:refnum<file>)  [unwired: 1 in, 4 out]
        n851 = Deny Access(7:w1355) -> (3:w1353:refnum<file>)  [unwired: 1 in, 2 out]
        n852 = Read from Binary File(5:0.0, 8:w1372, 9:w1351, 10:w1352, 11:w1376) -> (0:w1371:errorcluster, 2:w1369:dbl[], 3:w1374:refnum<file>)  [unwired: 2 out]
        n853 = Array To Cluster(array=w1369) -> (cluster=w1368:T32)
        n854 = Unbundle(w1368) -> ("[0]"=w1342:dbl, "[1]"=w1340:dbl, "[2]"=w1341:dbl, "[3]"=w1339:dbl, "[4]"=w1367:dbl, "[5]"=w1366:dbl)
        n855 = Close File(refnum=w1374, error in=w1371) -> (error out=→"Read cal error":errorcluster)  [unwired: 1 out]
        n856 = Multiply(x=w1366, y=w1363) -> (x*y=w1364:dbl)
        n857 = local write "T2 kappa_x (pN/nm)"(w1339) -> ()
        n858 = local write "T1 kappa_x (pN/nm)"(w1341) -> ()
        n859 = local write "T1 alpha_x (nm/V)"(w1342) -> ()
        n860 = local write "T2 alpha_x (nm/V)"(w1340) -> ()
        n861 = Read from Binary File(5:0.0, 9:w1351, 10:w1352, 11:w1353) -> (2:w1347:dbl[], 3:w1350:refnum<file>)  [unwired: 1 in, 3 out]
        n862 = Multiply(x=w1367, y=w1363) -> (x*y=w1365:dbl)
        n863 = local write "T1 offset_x (mV)"(w1365) -> ()
        n864 = local write "T2 offset_x (mV)"(w1364) -> ()
        n865 = Close File(refnum=w1350) -> ()  [unwired: 1 in, 2 out]
        n866 = Array Subset(array=w1347, index=3) -> (w1345:dbl[])  [unwired: 1 in]
        n867 = Index Array(array=w1347, index=0) -> (element=→"Offset file step size":dbl)
        n868 = Multiply(x=w1342, y=w1341) -> (x*y=w1337:dbl)
        n869 = Multiply(x=w1340, y=w1339) -> (x*y=w1338:dbl)
        n870 = Divide(x=w1338, y=w1337) -> (x/y=w1332:dbl)
        n871 = Decimate 1D Array(w1345) -> (w1335:dbl[], w1336:dbl[])  [unwired: 1 out]
        n872 = property on="B factor" class="DigNum (strict)"("Val(Sgnl)"=w1332) -> ()  [unwired: 2 in, 2 out]
        n873 = Bundle By Name(cluster="Offset Values", "Trap 1X offset"=w1335, "Trap 2X offset"=w1336) -> (w1343:T14)
        n874 = Multiply(x=w1336, y=w1332) -> (x*y=w1334:dbl[])
        n875 = Subtract(x=w1335, y=w1334) -> (x-y=w1333:dbl[])
        n876 = local write "Offset Values"(w1343) -> ()
        n877 = case shown="True" "Auto read offset\ncorrection" {
          tunnel: w1333 -> [_ w1385]
          frame False {
          }
          frame True {
            n878 = property on="Setpoint offset\nCorrection values" class="Arr (strict)"("Val(Sgnl)"=w1385) -> ()  [unwired: 2 in, 2 out]
          }
        }
      }
      event "Abort MCL Scan": Value Change {
        n879 = event-data() -> ()  [unwired: 7 out]
        n880 = local write "MCL Scanning"(FALSE ("MCL Scanning")) -> ()
        n881 = xnode "Read/Write Control"("FPGA VI Reference In"=w1390, "error in"=w1389, "Abort scan (MCL)"="Abort MCL Scan") -> ("error out"=w1388:errorcluster)  [unwired: 1 out]
      }
      event "Update Count (MCL)": Value Change {
        n882 = event-data() -> ()  [unwired: 7 out]
        n883 = xnode "Read/Write Control"("FPGA VI Reference In"=w1394, "error in"=w1393, "MCL count"="Update Count (MCL)") -> ("error out"=w1392:errorcluster)  [unwired: 1 out]
      }
      event "Phase adjust (MCL)", "+ phase (MCL)", "- phase (MCL)": Value Change {
        n884 = event-data() -> ()  [unwired: 7 out]
        n885 = Negate(x="Phase adjust (MCL)") -> (-x=w1403:i16)
        n886 = Select(t=w1403, s="- phase (MCL)", f="Phase adjust (MCL)") -> (s? t:f=w1401:i16)
        n887 = Or(x="- phase (MCL)", y="+ phase (MCL)") -> (x .or. y?=w1396:bool)
        n888 = xnode "Read/Write Control"("FPGA VI Reference In"=w1405, "error in"=w1404, "Phase count adjustment (MCL)"=w1401) -> ("FPGA VI Reference Out"=w1397:T20, "error out"=w1398:errorcluster)
        n889 = xnode "Read/Write Control"("FPGA VI Reference In"=w1397, "error in"=w1398, "+ phase (MCL)"=w1396) -> ("error out"=w1395:errorcluster)  [unwired: 1 out]
      }
      event "Abort AOD Scan": Value Change {
        n890 = event-data() -> ()  [unwired: 7 out]
        n891 = xnode "Read/Write Control"("FPGA VI Reference In"=w1409, "error in"=w1408, "Abort scan"="Abort AOD Scan") -> ("error out"=w1407:errorcluster)  [unwired: 1 out]
      }
      event "Continuous AOD Scanning": Value Change {
        n892 = event-data() -> ()  [unwired: 7 out]
        n893 = xnode "Read/Write Control"("FPGA VI Reference In"=w1413, "error in"=w1412, "Cont. Scan"="Continuous AOD Scanning") -> ("error out"=w1411:errorcluster)  [unwired: 1 out]
      }
      event "Index": Value Change {
        n894 = event-data() -> ()  [unwired: 7 out]
        n895 = call "Create new save file.vi"("Insert"="", "Ext"=".dat" ("string"), "Index In"="Index") -> ("Path Out"=→"Save file name":path, "Index Out"=w1414:dbl)
        "Save index" <- w1414
        n896 = local write "Index"(w1414) -> ()
      }
      event "AO1", "AO2": Value Change {
        w1429 = 10.0 ("y")
        w1428 = 32767.0 ("y")
        n897 = event-data() -> ()  [unwired: 7 out]
        n898 = local read "AO2"() -> (w1427:dbl)
        n899 = local read "AO1"() -> (w1424:dbl)
        n900 = Multiply(x=w1424, y=w1428) -> (x*y=w1423:dbl)
        n901 = Multiply(x=w1427, y=w1428) -> (x*y=w1426:dbl)
        n902 = Divide(x=w1423, y=w1429) -> (x/y=w1422:dbl)
        n903 = Divide(x=w1426, y=w1429) -> (x/y=w1425:dbl)
        n904 = To Word Integer(number=w1422) -> (16bit integer=w1430:i16)
        n905 = To Word Integer(number=w1425) -> (16bit integer=w1431:i16)
        n906 = xnode "Read/Write Control"("FPGA VI Reference In"=w1421, "error in"=w1420, "AO1"=w1430, "AO2"=w1431) -> ("error out"=w1419:errorcluster)  [unwired: 1 out]
      }
      event "Inject Top:": Value Change {
        n907 = event-data() -> ()  [unwired: 7 out]
        n908 = disable-structure shown="Enabled" {
          disable-tunnel: "Inject Top:" -> [w1433 w1473]
          frame Disabled {
            n909 = local read "Chemyx Syringe Pump Serial Port"() -> (w1434:refnum<visa-resource-name>)
            n910 = local read "Pump write delay (ms)"() -> (w1435:dbl)
            n911 = case shown="True" w1433 {
              tunnel: w1435 -> [w1441 w1455]
              tunnel: w1434 -> [w1438 w1454]
              frame False {
                n912 = flat-sequence {
                  tunnel: w1438 -> [w1442]
                  tunnel: [w1442] -> w1439
                  tunnel: w1441 -> [_]
                  tunnel: [w1445] -> w1440
                  tunnel: w1439 -> [w1445]
                  tunnel: w1440 -> [w1446]
                  tunnel: [w1446] -> w1436
                  tunnel: [w1448] -> w1437
                  tunnel: w1436 -> [w1448]
                  tunnel: w1437 -> [w1450]
                  frame #0 {
                    n913 = call "Write to pump.vi"("string"="enter pump1", "VISA resource name"=w1442) -> ()  [unwired: 1 out]
                  }
                  frame #1 {
                    n914 = Wait (ms)(milliseconds to wait="Pump pause delay (ms)") -> ()  [unwired: 1 out]
                  }
                  frame #2 {
                    n915 = call "Write to pump.vi"("string"="stop", "VISA resource name"=w1446) -> ()  [unwired: 1 out]
                  }
                  frame #3 {
                    n916 = Wait (ms)(milliseconds to wait=u32 500) -> ()  [unwired: 1 out]
                  }
                  frame #4 {
                    n917 = call "Write to pump.vi"("string"="stop", "VISA resource name"=w1450) -> ()  [unwired: 1 out]
                  }
                }
              }
              frame True {
                n918 = flat-sequence {
                  tunnel: w1454 -> [w1464]
                  tunnel: w1455 -> [w1459]
                  tunnel: w1455 -> [w1466]
                  tunnel: w1454 -> [w1467]
                  tunnel: [w1467] -> w1452
                  tunnel: [w1469] -> w1453
                  tunnel: w1452 -> [w1469]
                  tunnel: w1453 -> [w1471]
                  frame #0 {
                    n919 = local read "All Pump Parameters"() -> (w1458:T6)
                    n920 = Unbundle By Name(w1458) -> ("Pump 1"=w1465:T33)
                    n921 = call "Set pump parameters.vi"("Pump write delay (ms)"=w1459, "Volume (uL)"="Ch 2 Inject Volume (uL)", "Rate (uL/h)"="Ch 1 Inject Rate (ul/h)", "Units"=4.0, "Pump #"=1.0, "Pump Parameters In"=w1465, "VISA resource name"=w1464) -> ("Pump Parameters Out"=w1457:T33)  [unwired: 3 in]
                    n922 = Bundle By Name(cluster=w1458, "Pump 1"=w1457) -> (w1456:T6)
                    n923 = local write "All Pump Parameters"(w1456) -> ()
                  }
                  frame #1 {
                    n924 = Wait (ms)(milliseconds to wait=w1466) -> ()  [unwired: 1 out]
                  }
                  frame #2 {
                    n925 = call "Write to pump.vi"("string"="start", "VISA resource name"=w1467) -> ()  [unwired: 1 out]
                  }
                  frame #3 {
                    n926 = Wait (ms)(milliseconds to wait=u32 500) -> ()  [unwired: 1 out]
                  }
                  frame #4 {
                    n927 = call "Write to pump.vi"("string"="start", "VISA resource name"=w1471) -> ()  [unwired: 1 out]
                  }
                }
              }
            }
          }
          frame Enabled {
            n928 = call "hamilton_controller.vi"("Open?"=w1473, "valve"=enum16{"A", "B", "C", "D", "ALL"}."B", "action"=T21."MOVE VALVE") -> ()  [unwired: 8 in, 1 out]
          }
        }
      }
      event "Main:": Value Change {
        n929 = event-data() -> ()  [unwired: 7 out]
        n930 = disable-structure shown="Disabled" {
          disable-tunnel: "Main:" -> [_ w1517]
          frame Disabled {
            n931 = local read "Pump write delay (ms)"() -> (w1478:dbl)
            n932 = case shown="False" w1479 {
              tunnel: w1478 -> [w1485 w1499]
              tunnel: "Chemyx Syringe Pump Serial Port" -> [w1482 w1498]
              frame False {
                n933 = flat-sequence {
                  tunnel: w1482 -> [w1486]
                  tunnel: [w1486] -> w1483
                  tunnel: w1485 -> [_]
                  tunnel: [w1489] -> w1484
                  tunnel: w1483 -> [w1489]
                  tunnel: w1484 -> [w1490]
                  tunnel: [w1490] -> w1480
                  tunnel: [w1492] -> w1481
                  tunnel: w1480 -> [w1492]
                  tunnel: w1481 -> [w1494]
                  frame #0 {
                    n934 = call "Write to pump.vi"("string"="enter pump3", "VISA resource name"=w1486) -> ()  [unwired: 1 out]
                  }
                  frame #1 {
                    n935 = local read "Pump pause delay (ms)"() -> (w1488:u32)
                    n936 = Wait (ms)(milliseconds to wait=w1488) -> ()  [unwired: 1 out]
                  }
                  frame #2 {
                    n937 = call "Write to pump.vi"("string"="stop", "VISA resource name"=w1490) -> ()  [unwired: 1 out]
                  }
                  frame #3 {
                    n938 = Wait (ms)(milliseconds to wait=u32 0) -> ()  [unwired: 1 out]
                  }
                  frame #4 {
                    n939 = call "Write to pump.vi"("string"="stop", "VISA resource name"=w1494) -> ()  [unwired: 1 out]
                  }
                }
              }
              frame True {
                n940 = flat-sequence {
                  tunnel: w1498 -> [w1508]
                  tunnel: w1499 -> [w1503]
                  tunnel: w1499 -> [w1510]
                  tunnel: w1498 -> [w1511]
                  tunnel: [w1511] -> w1496
                  tunnel: [w1514] -> w1497
                  tunnel: w1496 -> [w1514]
                  tunnel: w1497 -> [w1515]
                  frame #0 {
                    n941 = local read "All Pump Parameters"() -> (w1502:T6)
                    n942 = Unbundle By Name(w1502) -> ("Pump 3"=w1509:T33)
                    n943 = call "Set pump parameters.vi"("Pump write delay (ms)"=w1503, "Volume (uL)"="Ch 3 Inject Volume (uL)", "Rate (uL/h)"="Ch 3 Inject Rate (ul/h)", "Units"=4.0, "Pump #"=3.0, "Pump Parameters In"=w1509, "VISA resource name"=w1508) -> ("Pump Parameters Out"=w1501:T33)  [unwired: 3 in]
                    n944 = Bundle By Name(cluster=w1502, "Pump 3"=w1501) -> (w1500:T6)
                    n945 = local write "All Pump Parameters"(w1500) -> ()
                  }
                  frame #1 {
                    n946 = Wait (ms)(milliseconds to wait=w1510) -> ()  [unwired: 1 out]
                  }
                  frame #2 {
                    n947 = call "Write to pump.vi"("string"="start", "VISA resource name"=w1511) -> ()  [unwired: 1 out]
                  }
                  frame #3 {
